vi "lib Graph Pixel Offset.vi"(6 "X Pix Offset":i32=8, 8 "error in (no error)":errorcluster, 9 "Y Pix Offset":i32=8, 10 "XY":cluster{"X":dbl, "Y":dbl}, 11 "Graph":refnum<vi>) -> (0 "error out":errorcluster, 2 "XY Offset":cluster{"X":dbl, "Y":dbl}, 3 "Graph out":refnum<vi>)   [LabVIEW 2014]
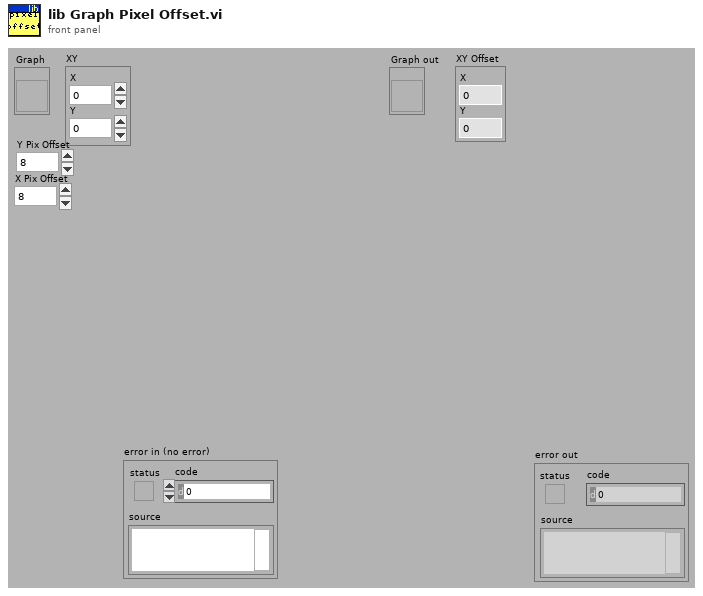
[diagram p1: front panel]
types:
  T1 = typedef "LVPoint32TypeDef.ctl" = cluster{"Horizontal":i32, "Vertical":i32}
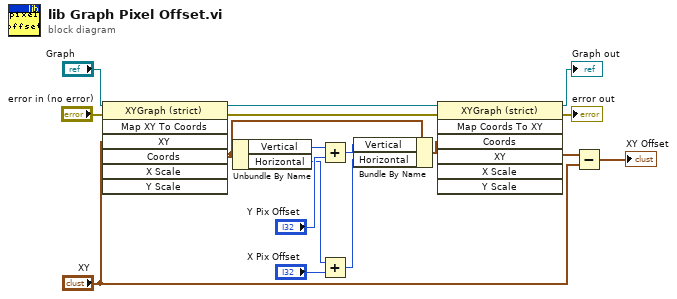
[diagram p0: block diagram]
diagram:
  n1 = invoke class="XYGraph (strict)" method="Map XY To Coords"(reference="Graph", error in="error in (no error)", "XY"="XY") -> (reference out=w17:refnum<vi>, error out=w2:errorcluster, "Coords"=w12:T1)  [unwired: 4 in, 4 out]
  n2 = Unbundle By Name(w12) -> ("Vertical"=w16:i32, "Horizontal"=w7:i32)
  n3 = Add(x=w16, y="Y Pix Offset") -> (x+y=w14:i32)
  n4 = Add(x=w7, y="X Pix Offset") -> (x+y=w5:i32)
  n5 = Bundle By Name(cluster=w12, "Vertical"=w14, "Horizontal"=w5) -> (w13:T1)
  n6 = invoke class="XYGraph (strict)" method="Map Coords To XY"(reference=w17, error in=w2, "Coords"=w13) -> (reference out=→"Graph out":refnum<vi>, error out=→"error out":errorcluster, "XY"=w9:cluster{"X":dbl, "Y":dbl})  [unwired: 4 in, 4 out]
  n7 = Subtract(x=w9, y="XY") -> (x-y=→"XY Offset":cluster{"X":dbl, "Y":dbl})
